vi "WLM.vi"(1 "In":variant, 2 "Mode":u32(ring) items=["Open", "Close", "Begin", "End", "Get", "Set"]) -> (0 "Out":variant)   [LabVIEW 2014]
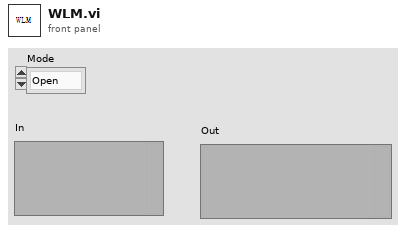
[diagram p1: front panel]
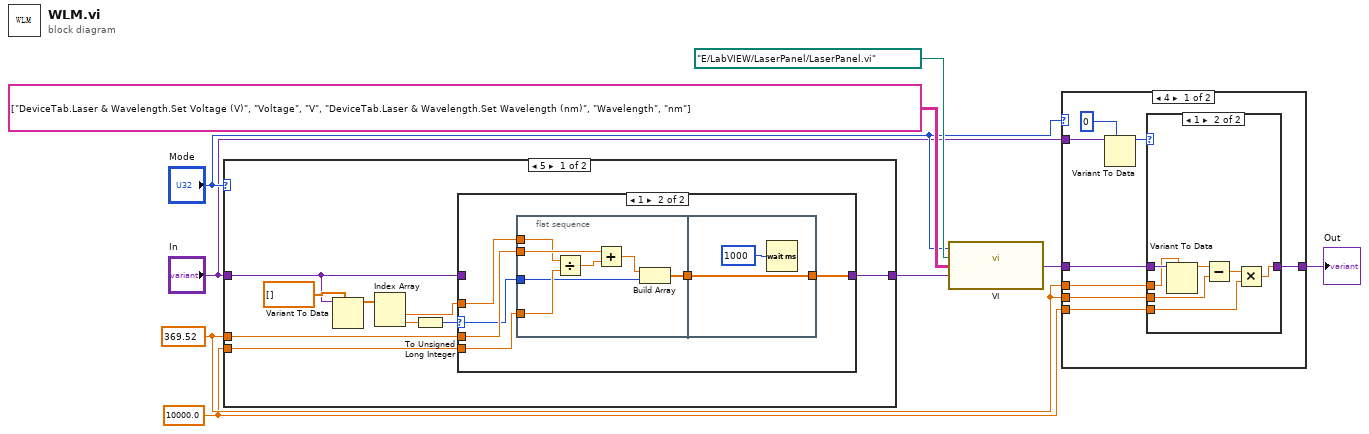
[diagram p0: block diagram]
diagram:
  w2 = 10000.0 ("y")
  w3 = 369.52
  n1 = case shown="5" "Mode" {
    tunnel: [w18 w35] -> w8
    tunnel: "In" -> [w10 w35]
    tunnel: w3 -> [w17 _]
    tunnel: w2 -> [w16 _]
    frame 5 {
      n2 = Variant To Data(type=dbl[] [] ("appended array"), Variant=w10) -> (data=w14:dbl[])  [unwired: 1 in, 1 out]
      n3 = Index Array(array=w14) -> (element #1=w13:dbl, element #2=w12:dbl)  [unwired: 2 in]
      n4 = To Unsigned Long Integer(number=w12) -> (unsigned 32bit integer=w11:u32)
      n5 = case shown="1" w11 {
        selector: w11 -> [_ w22]
        tunnel: [w19 w20] -> w18
        tunnel: w17 -> [_ w25]
        tunnel: w16 -> [_ w24]
        tunnel: w13 -> [_ w23]
        tunnel: w10 -> [w19 _]
        frame Default {
        }
        frame 1 {
          n6 = flat-sequence {
            tunnel: w25 -> [w31]
            tunnel: w24 -> [w30]
            tunnel: w23 -> [w29]
            tunnel: w22 -> [w27]
            tunnel: [w26] -> w21
            tunnel: [w33] -> w20
            tunnel: w21 -> [w33]
            frame #0 {
              n7 = Divide(x=w29, y=w30) -> (x/y=w32:dbl)
              n8 = Add(x=w31, y=w32) -> (x+y=w28:dbl)
              n9 = Build Array(w28, w27) -> (w26:dbl[])
            }
            frame #1 {
              n10 = Wait (ms)(milliseconds to wait=u32 1000) -> ()  [unwired: 1 out]
            }
          }
        }
      }
    }
    frame Default {
    }
  }
  n11 = call "VI.vi"("In"=w8, "Names"=string[][] [["DeviceTab.Laser & Wavelength.Set Voltage (V)", "Voltage", "V"], ["DeviceTab.Laser & Wavelength.Set Wavelength (nm)", "Wavelength", "nm"]], "Path"=path "E:/LabVIEW/LaserPanel/LaserPanel.vi", "Mode"="Mode") -> ("Out"=w9:variant)
  n12 = case shown="4" "Mode" {
    tunnel: w9 -> [w42 w52]
    tunnel: [w39 w52] -> w4
    tunnel: w3 -> [w43 _]
    tunnel: w3 -> [w41 _]
    tunnel: w2 -> [w40 _]
    tunnel: "In" -> [w37 _]
    frame 4 {
      n13 = Variant To Data(type=u32 0, Variant=w37) -> (data=w36:u32)  [unwired: 1 in, 1 out]
      n14 = case shown="1" w36 {
        tunnel: w43 -> [_ w51]
        tunnel: w42 -> [w44 w50]
        tunnel: w41 -> [_ w49]
        tunnel: w40 -> [_ w46]
        tunnel: [w44 w45] -> w39
        frame Default {
        }
        frame 1 {
          n15 = Variant To Data(type=w49, Variant=w50) -> (data=w48:dbl)  [unwired: 1 in, 1 out]
          n16 = Subtract(x=w48, y=w51) -> (x-y=w47:dbl)
          n17 = Multiply(x=w47, y=w46) -> (x*y=w45:dbl)
        }
      }
    }
    frame Default {
    }
  }
  "Out" <- w4
